vi "pco.camera_Live_ConvertSettings_Example_IMAQ.vi"() -> ()   [LabVIEW 2019]
doc: "A short program to demonstrate the fundamentals of control and image acquision with the pco.camera series. The program records a sequence of images, with \"live\" updating, until the \"StopRecording\" button is pressed. Use ctrl-H for more help on the individual controls and indicators.\n\nCopyright 2004, 2010 The Cooke Corporation."
uses:
  pco.camera/Camera.lvclass
  pco.sdk/TimingControl/TimingControl.lvlib
panel:
  in  "settingsChanged":bool
  in  "Trigger":bool
  in  "LUT File":path
  in  "data_format":T1(ring)=enum."RGBA8"
  out "Image":T2(plugin-control)
  in  "Auto Range":bool
  out "rawImage":u16[][](array[numeric])
  in  "iContrast [%]":i32 min=-100 max=99 step=1
  in  "Gamma":dbl=1.0 min=0.01 max=10.0 step=0.01 format="%.2f"
  in  "whiteBalance":bool
  in  "iScale_max":u16=60000 step=1
  in  "iScale_min":u16=200 step=1
  in  "Image Index":u32 max=9
  out "Recorded Images":u32
  in  "TriggerMode":T3(ring)
  in  "Quit":bool
  out "Error":errorcluster {"code" format="%x"}
  in  "Stop Record":bool
  out "Recording On":bool
  in  "roiY1":u64=2 min=1 max=2160 step=1
  in  "roiX1":u64=2 min=1 max=2560 step=1
  in  "roiY0":u64=1 min=1 max=2159 step=1
  in  "roiX0":u64=1 min=1 max=2559 step=1
  out "Image Height":u64
  out "Image Width":u64
  in  "dwImgCount":u32=10 caption="Required Number of Images" max=2397
  in  "Exposure Time [s]":dbl=0.010000000000000002 min=0.0005 max=2.0 step=0.001
  # "This example demonstrates the image acquisition with one camera in ring buffer mode together with a live display of the latest images during record. After record is stopped, the images can be addressed by index.\nAdditionally the image convert settings can be adjusted at any time\nNote that this example will not be fail save, i.e. doesnt react on errors, just handles them forward to the end\n\nUsage:\nSelect your required image count and the camera setup before you start the program.\nOnce started, the camera class will be initialized and images will be recorded and displayed automatically\nYou can stop the images by pressing stop record.\nAfter stopped, the image at the selected index will be read out\nTo finish the program click on quit application, this will force an exit of the camera class\nYou can change your required ROI after and also during the record."
  # "pco.labview"
  # "Camera Setup"
  # "Recording Control"
  # "Parameters for image readout"
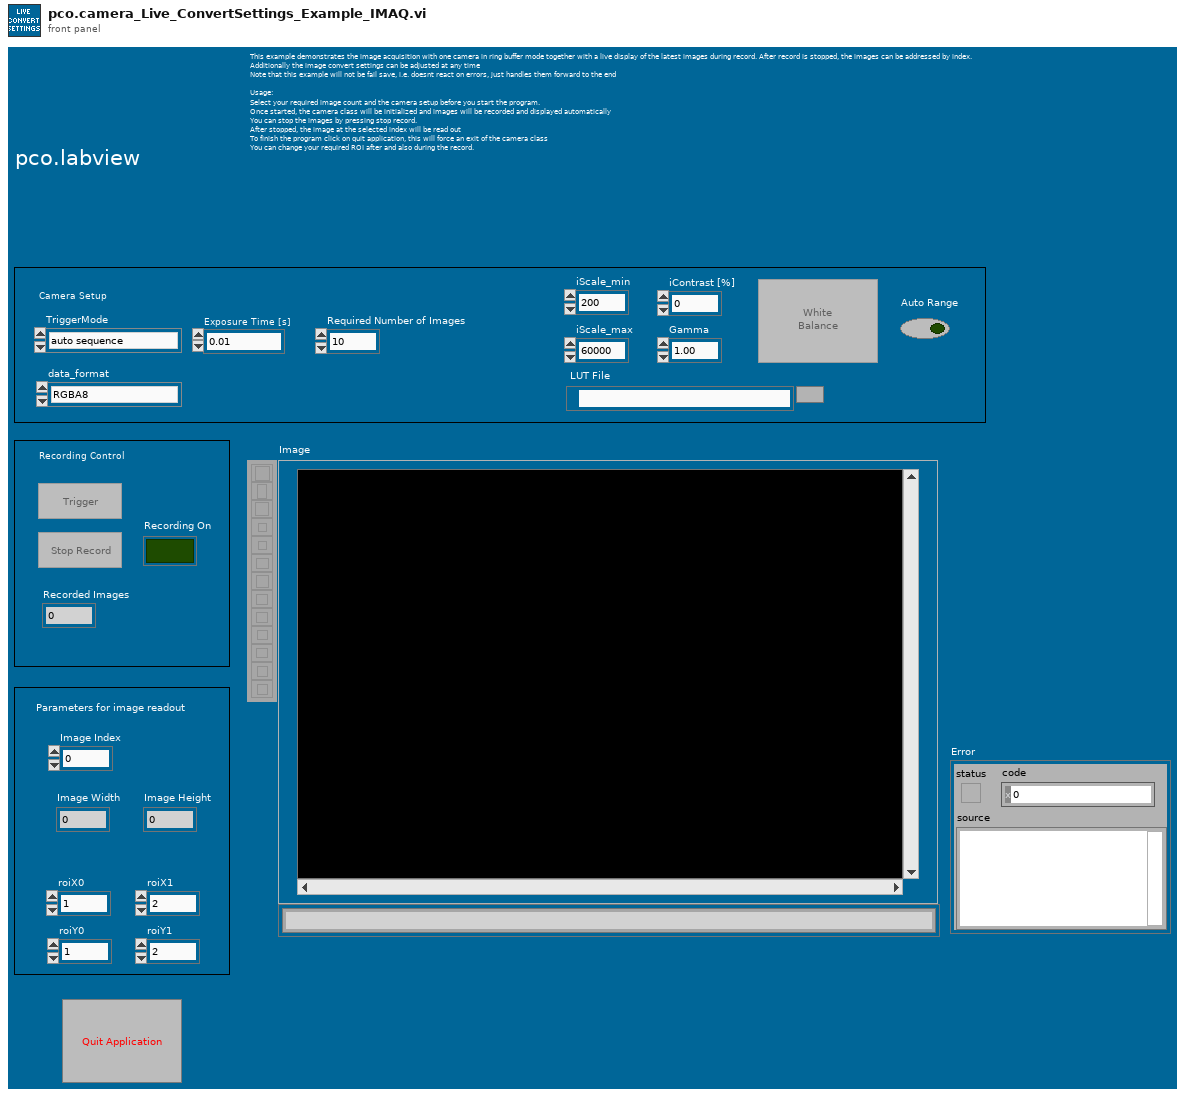
[diagram p1: front panel]
types:
  T1 = enum16{"Undefined", "Mono8", "Mono16", "BGRA8", "RGBA8", "BGRA16", "RGBA16", "CompressedMono8"}
  T2 = typedef "IMAQ Image.ctl" = refnum<image>
  T3 = enum16{"auto sequence", "software trigger", "external exposure start", "external exposure control"}
  T4 = enum16{"sequence", "sequence non blocking", "ring buffer", "fifo", "sequence_dpcore", "sequence_non_blocking_dpcore", "ring_buffer_dpcore", "fifo_dpcore", "tif", "multitif", "pcoraw", "b16", "dicom", "multidicom"}
  T5 = enum8{"Enabled", "Disabled", "Disabled and Grayed Out"}
  T6 = cluster{"serial":u32, "type":u16, "sub_type":u16, "interface_type":u16, "min_exposure_time_s":dbl, "max_exposure_time_s":dbl, "min_exposure_step_s":dbl, "min_delay_time_s":dbl, "max_delay_time_s":dbl, "min_delay_step_s":dbl, "min_width":u64, "min_height":u64, "max_width":u64, "max_height":u64, "roi_step_horz":u64, "roi_step_vert":u64, "roi_symmetric_horz":bool, "roi_symmetric_vert":bool, "has_timestamp_mode":bool, "has_timestamp_mode_ascii_only":bool, "pixelrate_vec":u32[], "has_acquire_mode":bool, "has_ext_acquire_mode":bool, "has_metadata_mode":bool, "has_ram":bool, "binning_horz_vec":u16[], "binning_vert_vec":u16[]}
  T7 = typedef "Image Type" = u32
  T8 = typedef "Camera.lvclass/binning.ctl" = cluster{"vert":u16, "horz":u16}
  T9 = cluster{"exposure_time_s":dbl, "delay_time_s":dbl, "roi":cluster{"x0":u64, "y0":u64, "x1":u64, "y1":u64}, "timestamp_mode":u16, "pixelrate":u32, "trigger_mode":u16, "acquire_mode":u16, "metadata_mode":u16, "noisefilter_mode":u16, "binning":T8}
  T10 = cluster{"sharpen":bool, "adaptive_sharpen":bool, "flip_vertical":bool, "auto_minmax":bool, "min_limit":u16, "max_limit":u16, "gamma":dbl, "contrast":i32, "pco_debayer_algorithm":bool, "color_temperature":i32, "color_saturation":i32, "color_vibrance":i32, "color_tint":i32, "lut_file":path}
  T11 = typedef "Color (U64)" = cluster{"Plane 3 (Blue)":u16, "Plane 2 (Green)":u16, "Plane 1 (Red)":u16, "Plane 4 (alpha)":u16}
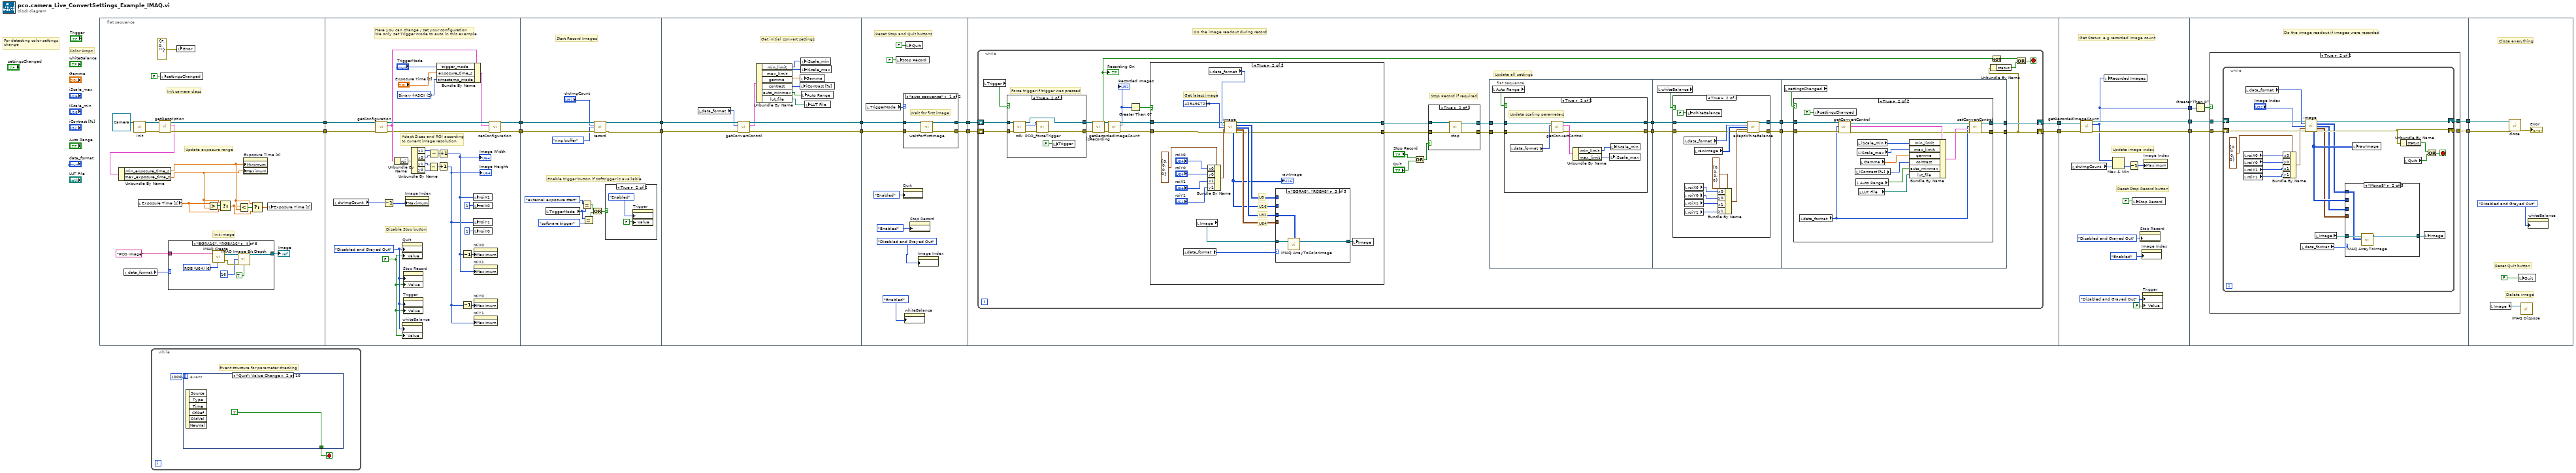
[diagram p0: block diagram]
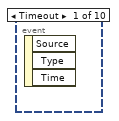
[diagram p2: hidden frame]
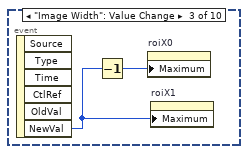
[diagram p3: hidden frame]
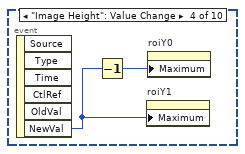
[diagram p4: hidden frame]
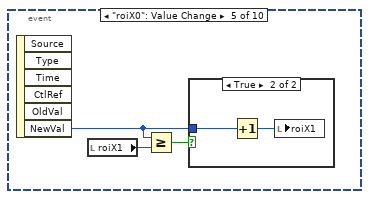
[diagram p5: hidden frame]
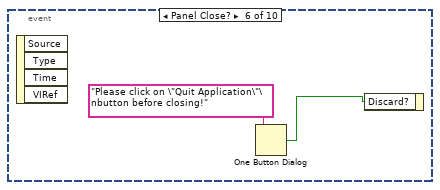
[diagram p7: hidden frame]
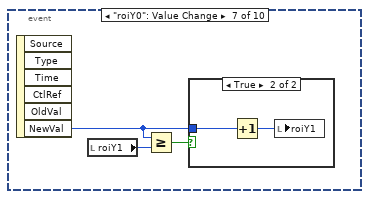
[diagram p8: hidden frame]
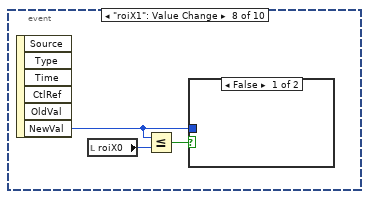
[diagram p10: hidden frame]
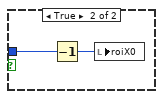
[diagram p11: hidden frame]
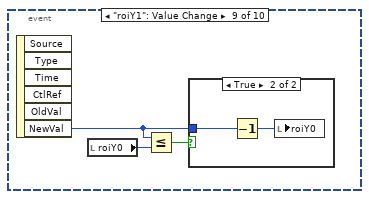
[diagram p12: hidden frame]
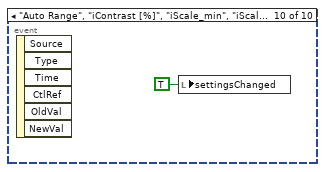
[diagram p14: hidden frame]
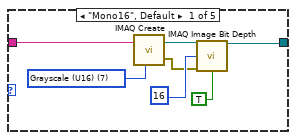
[diagram p15: hidden frame]
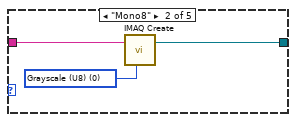
[diagram p16: hidden frame]
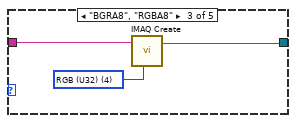
[diagram p17: hidden frame]
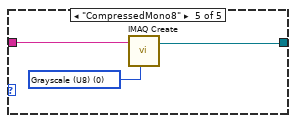
[diagram p18: hidden frame]
diagram:
  # "For detecting color settings\nchange"
  # "Color Props"
  n1 = flat-sequence {
    tunnel: [w24] -> w7
    tunnel: [w23] -> w6
    tunnel: [w63] -> w17
    tunnel: [w67] -> w16
    tunnel: w7 -> [w62]
    tunnel: w6 -> [w61]
    tunnel: w17 -> [w97]
    tunnel: w16 -> [w98]
    tunnel: [w94] -> w11
    tunnel: [w95] -> w8
    tunnel: w11 -> [w111]
    tunnel: [w106] -> w10
    tunnel: [w112] -> w9
    tunnel: w8 -> [w102]
    tunnel: w10 -> [w119]
    tunnel: w9 -> [w120]
    tunnel: [w118] -> w15
    tunnel: [w115] -> w2
    tunnel: w15 -> [w133]
    tunnel: [w132] -> w14
    tunnel: [w131] -> w5
    tunnel: w2 -> [w130]
    tunnel: w14 -> [w280]
    tunnel: [w278] -> w13
    tunnel: w5 -> [w273]
    tunnel: [w272] -> w4
    tunnel: [w271] -> w1
    tunnel: w13 -> [w289]
    tunnel: [w288] -> w12
    tunnel: w4 -> [w287]
    tunnel: [w286] -> w3
    tunnel: w1 -> [w284]
    tunnel: w12 -> [w337]
    tunnel: w3 -> [w334]
    frame #0 {
      # "Init image"
      # "Init camera class"
      # "Update exposure range"
      n2 = local read "data_format"() -> (w19:T1)
      n3 = call-dynamic "init.vi"("Camera in"=refnum<class "Camera.lvclass"> refnum) -> ("Camera out"=w25:refnum<class "Camera.lvclass">, "error out"=w26:errorcluster)  [unwired: 8 in]
      n4 = local read "Exposure Time [s]"() -> (w34:dbl)
      n5 = call-dynamic "getDescription.vi"("error in (no error)"=w26, "Camera in"=w25) -> ("error out"=w23:errorcluster, "description"=w22:T6, "Camera out"=w24:refnum<class "Camera.lvclass">)  [unwired: 7 in]
      n6 = Unbundle By Name(w22) -> ("min_exposure_time_s"=w21:dbl, "max_exposure_time_s"=w20:dbl)
      n7 = local write "settingsChanged"(FALSE ("settingsChanged")) -> ()
      n8 = case shown="\"BGRA16\", \"RGBA16\"" w19 {
        tunnel: "PCO Image" ("Image Name") -> [w41 w45 w47 w54 w57]
        tunnel: [w36 w43 w46 w49 w56] -> w27
        frame "Mono16", Default {
          w42 = T7 7 items=["Grayscale (U8)", "Grayscale (I16)", "Grayscale (SGL)", "Complex (CSG)", "RGB (U32)", "HSL (U32)", "RGB (U64)", "Grayscale (U16)"] ("Image Type")
          n9 = call "IMAQ Create"("Image Name"=w41, "Image Type"=w42) -> ("New Image"=w38:T2, "error out"=w37:errorcluster)  [unwired: 3 in]
          n10 = call "IMAQ Image Bit Depth"("Image"=w38, "Bit Depth (0)"=u32 16, "error in (no error)"=w37, "Get/Set Bit Depth? (Set)"=TRUE) -> ("Image Out"=w36:T2)  [unwired: 9 in, 2 out]
        }
        frame "Mono8" {
          w44 = T7 0 items=["Grayscale (U8)", "Grayscale (I16)", "Grayscale (SGL)", "Complex (CSG)", "RGB (U32)", "HSL (U32)", "RGB (U64)", "Grayscale (U16)"] ("Image Type")
          n11 = call "IMAQ Create"("Image Name"=w45, "Image Type"=w44) -> ("New Image"=w43:T2)  [unwired: 3 in, 1 out]
        }
        frame "BGRA8", "RGBA8" {
          w48 = T7 4 items=["Grayscale (U8)", "Grayscale (I16)", "Grayscale (SGL)", "Complex (CSG)", "RGB (U32)", "HSL (U32)", "RGB (U64)", "Grayscale (U16)"] ("Image Type")
          n12 = call "IMAQ Create"("Image Name"=w47, "Image Type"=w48) -> ("New Image"=w46:T2)  [unwired: 3 in, 1 out]
        }
        frame "BGRA16", "RGBA16" {
          w55 = T7 6 items=["Grayscale (U8)", "Grayscale (I16)", "Grayscale (SGL)", "Complex (CSG)", "RGB (U32)", "HSL (U32)", "RGB (U64)", "Grayscale (U16)"] ("Image Type")
          n13 = call "IMAQ Create"("Image Name"=w54, "Image Type"=w55) -> ("New Image"=w51:T2, "error out"=w50:errorcluster)  [unwired: 3 in]
          n14 = call "IMAQ Image Bit Depth"("Image"=w51, "Bit Depth (0)"=u32 16, "error in (no error)"=w50, "Get/Set Bit Depth? (Set)"=TRUE) -> ("Image Out"=w49:T2)  [unwired: 9 in, 2 out]
        }
        frame "CompressedMono8" {
          w58 = T7 0 items=["Grayscale (U8)", "Grayscale (I16)", "Grayscale (SGL)", "Complex (CSG)", "RGB (U32)", "HSL (U32)", "RGB (U64)", "Grayscale (U16)"] ("Image Type")
          n15 = call "IMAQ Create"("Image Name"=w57, "Image Type"=w58) -> ("New Image"=w56:T2)  [unwired: 3 in, 1 out]
        }
      }
      "Image" <- w27
      n16 = local write "Error"(errorcluster {"status"=FALSE, "code"=0, "source"=""} ("error IO")) -> ()
      n17 = Greater?(x=w34, y=w20) -> (0:w35:bool)
      n18 = Select(t=w20, s=w35, f=w34) -> (s? t:f=w32:dbl)
      n19 = Less?(x=w32, y=w21) -> (x < y?=w33:bool)
      n20 = property on="Exposure Time [s]" class="DigNum (strict)"("Minimum"=w21, "Maximum"=w20) -> ()  [unwired: 2 in, 2 out]
      n21 = Select(t=w21, s=w33, f=w32) -> (s? t:f=w31:dbl)
      n22 = local write "Exposure Time [s]"(w31) -> ()
    }
    frame #1 {
      w73 = u16 2 items=["OFF", "Binary", "Binary+ASCII", "ASCII"] ("wTimeStampMode")
      w59 = FALSE ("Stop")
      w60 = T5."Disabled and Grayed Out" ("Disabled")
      # "Disable Stop button"
      # "Adapt Sizes and ROI according\nto current image resolution"
      # "Here you can change / set your configuration\nWe only set Trigger mode to auto in this example"
      n23 = local read "dwImgCount"() -> (w74:u32)
      n24 = call-dynamic "getConfiguration.vi"("error in (no error)"=w61, "Camera in"=w62) -> ("error out"=w68:errorcluster, "configuration"=w79:T9, "Camera out"=w70:refnum<class "Camera.lvclass">)  [unwired: 7 in]
      n25 = Decrement(x=w74) -> (x-1=w64:u32)
      n26 = Unbundle By Name(w79) -> ("roi"=w80:cluster{"x0":u64, "y0":u64, "x1":u64, "y1":u64})
      n27 = property on="Quit" class="Bool (strict)"("DisabledEnum"=w60, "Value"=w59) -> ()  [unwired: 2 in, 2 out]
      n28 = property on="whiteBalance" class="Bool (strict)"("DisabledEnum"=w60, "Value"=w59) -> ()  [unwired: 2 in, 2 out]
      n29 = property on="Stop Record" class="Bool (strict)"("DisabledEnum"=w60, "Value"=w59) -> ()  [unwired: 2 in, 2 out]
      n30 = property on="Trigger" class="Bool (strict)"("DisabledEnum"=w60, "Value"=w59) -> ()  [unwired: 2 in, 2 out]
      n31 = property on="Image Index" class="DigNum (strict)"("Maximum"=w64) -> ()  [unwired: 2 in, 2 out]
      n32 = Unbundle By Name(w80) -> ("x1"=w82:u64, "x0"=w81:u64, "y1"=w84:u64, "y0"=w83:u64)
      n33 = Subtract(x=w84, y=w83) -> (x-y=w86:u64)
      n34 = Subtract(x=w82, y=w81) -> (x-y=w85:u64)
      n35 = Bundle By Name(cluster=w79, "trigger_mode"="TriggerMode", "exposure_time_s"="Exposure Time [s]", "timestamp_mode"=w73) -> (w69:T9)
      n36 = Increment(x=w86) -> (x+1=w65:u64)
      "Image Height" <- w65
      n37 = Increment(x=w85) -> (x+1=w66:u64)
      "Image Width" <- w66
      n38 = Decrement(x=w66) -> (x-1=w77:u64)
      n39 = Decrement(x=w65) -> (x-1=w78:u64)
      n40 = local write "roiX1"(w66) -> ()
      n41 = local write "roiX0"(u64 1 ("roiY0")) -> ()
      n42 = local write "roiY1"(w65) -> ()
      n43 = local write "roiY0"(u64 1 ("roiY0")) -> ()
      n44 = property on="roiX0" class="DigNum (strict)"("Maximum"=w77) -> ()  [unwired: 2 in, 2 out]
      n45 = property on="roiX1" class="DigNum (strict)"("Maximum"=w66) -> ()  [unwired: 2 in, 2 out]
      n46 = property on="roiY0" class="DigNum (strict)"("Maximum"=w78) -> ()  [unwired: 2 in, 2 out]
      n47 = property on="roiY1" class="DigNum (strict)"("Maximum"=w65) -> ()  [unwired: 2 in, 2 out]
      n48 = call-dynamic "setConfiguration.vi"("error in (no error)"=w68, "configuration"=w69, "Camera in"=w70) -> ("error out"=w67:errorcluster, "Camera out"=w63:refnum<class "Camera.lvclass">)  [unwired: 7 in]
    }
    frame #2 {
      # "Enable trigger button if softtrigger is available"
      # "Start Record Images"
      n49 = local read "TriggerMode"() -> (w92:T3)
      n50 = Equal?(x=T3."external exposure start" ("TriggerMode"), y=w92) -> (x = y?=w89:bool)
      n51 = Equal?(x=w92, y=T3."software trigger" ("TriggerMode")) -> (x = y?=w88:bool)
      n52 = Or(x=w89, y=w88) -> (x .or. y?=w90:bool)
      n53 = call-dynamic "record.vi"("Camera in"=w97, "num_images"="dwImgCount", "record_mode"=T4."ring buffer", "error in (no error)"=w98) -> ("Camera out"=w95:refnum<class "Camera.lvclass">, "error out"=w94:errorcluster)  [unwired: 10 in]
      n54 = case shown="True" w90 {
        frame False {
        }
        frame True {
          n55 = property on="Trigger" class="Bool (strict)"("DisabledEnum"=T5."Enabled" ("Disabled"), "Value"=FALSE ("Trigger")) -> ()  [unwired: 2 in, 2 out]
        }
      }
    }
    frame #3 {
      # "Get initial convert settings"
      n56 = local read "data_format"() -> (w101:T1)
      n57 = call-dynamic "getConvertControl.vi"("error in (no error)"=w111, "data_format"=w101, "Camera in"=w102) -> ("error out"=w106:errorcluster, "convert_control"=w110:T10, "Camera out"=w112:refnum<class "Camera.lvclass">)  [unwired: 6 in]
      n58 = Unbundle By Name(w110) -> ("min_limit"=w108:u16, "max_limit"=w107:u16, "gamma"=w109:dbl, "contrast"=w105:i32, "auto_minmax"=w104:bool, "lut_file"=w103:path)
      n59 = local write "iContrast [%]"(w105) -> ()
      n60 = local write "Gamma"(w109) -> ()
      n61 = local write "iScale_min"(w108) -> ()
      n62 = local write "iScale_max"(w107) -> ()
      n63 = local write "Auto Range"(w104) -> ()
      n64 = local write "LUT File"(w103) -> ()
    }
    frame #4 {
      # "Reset Stop and Quit buttons"
      n65 = local read "TriggerMode"() -> (w113:T3)
      n66 = local write "Stop Record"(FALSE ("Stop Record")) -> ()
      n67 = case shown="\"auto sequence\"" w113 {
        tunnel: w120 -> [w127 w129]
        tunnel: w119 -> [w126 w128]
        tunnel: [w125 w128] -> w118
        tunnel: [w124 w129] -> w115
        frame "auto sequence" {
          # "Wait for first image"
          n68 = call-dynamic "waitForFirstImage.vi"("error in (no error)"=w126, "Camera in"=w127) -> ("error out"=w125:errorcluster, "Camera out"=w124:refnum<class "Camera.lvclass">)  [unwired: 8 in]
        }
        frame Default {
          # "Don't wait \nif we trigger"
        }
      }
      n69 = property on="Quit" class="Bool (strict)"("DisabledEnum"=T5."Enabled" ("Disabled")) -> ()  [unwired: 2 in, 2 out]
      n70 = property on="whiteBalance" class="Bool (strict)"("DisabledEnum"=T5."Enabled" ("Disabled")) -> ()  [unwired: 2 in, 2 out]
      n71 = local write "Quit"(FALSE ("Stop")) -> ()
      n72 = property on="Stop Record" class="Bool (strict)"("DisabledEnum"=T5."Enabled" ("Disabled")) -> ()  [unwired: 2 in, 2 out]
      n73 = property on="Image Index" class="DigNum (strict)"("DisabledEnum"=T5."Disabled and Grayed Out" ("Disabled")) -> ()  [unwired: 2 in, 2 out]
    }
    frame #5 {
      # "Do the image readout during record"
      n74 = while {
        shift-right: [w143] -> w132
        shift-left: w133 -> [w146]
        shift-right: [w149] -> w131
        shift-left: w130 -> [w147]
        stop <- w161 stop-if-true
        # "Stop Record if required"
        # "Force trigger if trigger was pressed"
        # "Update all settings"
        n75 = local read "Trigger"() -> (w148:bool)
        n76 = case shown="True" w148 {
          tunnel: w147 -> [w205 w210]
          tunnel: w146 -> [w204 w209]
          tunnel: [w205 w208] -> w145
          tunnel: [w204 w207] -> w144
          frame False {
          }
          frame True {
            n77 = call-dynamic "sdk.vi"("Camera in"=w210, "error in (no error)"=w209) -> ("Camera out"=w208:refnum<class "Camera.lvclass">, "sdk"=w211:u64, "error out"=w212:errorcluster)  [unwired: 11 in]
            n78 = call "PCO_ForceTrigger.vi"("error in (no error)"=w212, "ph"=w211) -> ("error out"=w207:errorcluster)  [unwired: 6 in, 3 out]
            n79 = local write "Trigger"(FALSE ("Trigger")) -> ()
          }
        }
        n80 = call-dynamic "isRecording.vi"("Camera in"=w145, "error in (no error)"=w144) -> ("Camera out"=w157:refnum<class "Camera.lvclass">, "recording"=w159:bool, "error out"=w156:errorcluster)  [unwired: 11 in]
        "Recording On" <- w159
        n81 = call-dynamic "getRecordedImageCount.vi"("Camera in"=w157, "error in (no error)"=w156) -> ("Camera out"=w154:refnum<class "Camera.lvclass">, "recorded_image_count"=w142:u32, "error out"=w155:errorcluster)  [unwired: 11 in]
        "Recorded Images" <- w142
        n82 = Greater Than 0?(x=w142) -> (x > 0?=w141:bool)
        n83 = case shown="True" w141 {
          tunnel: w155 -> [w168 w181]
          tunnel: w154 -> [w169 w172]
          tunnel: [w168 w170] -> w137
          tunnel: [w169 w171] -> w136
          frame False {
          }
          frame True {
            # "U64"
            # "U32"
            # "U8"
            # "U16"
            # "Get latest image"
            n84 = local read "data_format"() -> (w173:T1)
            n85 = local read "Image"() -> (w178:T2)
            n86 = Bundle By Name(cluster=cluster{"x0":u64, "y0":u64, "x1":u64, "y1":u64} {"x0"=0, "y0"=0, "x1"=0, "y1"=0} ("roi"), "x0"="roiX0", "y0"="roiY0", "x1"="roiX1", "y1"="roiY1") -> (w184:cluster{"x0":u64, "y0":u64, "x1":u64, "y1":u64})
            n87 = local read "data_format"() -> (w180:T1)
            n88 = call-dynamic "image.vi"("Camera in"=w172, "data_format"=w180, "image_index"=u32 4294967295 ("dwImgIdx"), "roi"=w184, "error in (no error)"=w181) -> ("Camera out"=w171:refnum<class "Camera.lvclass">, "image (U8)"=w175:u8[][], "image (U32)"=w176:u32[][], "image (U64)"=w177:T11[][], "raw_image (U16)"=w174:u16[][], "error out"=w170:errorcluster)  [unwired: 3 in, 2 out]
            "rawImage" <- w174
            n89 = case shown="\"BGRA8\", \"RGBA8\"" w173 {
              tunnel: w178 -> [w191 w194 w197 w200 w203]
              tunnel: [w189 w192 w196 w198 w202] -> w179
              tunnel: w177 -> [_ _ _ w199 _]
              tunnel: w176 -> [_ _ w195 _ _]
              tunnel: w175 -> [_ w193 _ _ w201]
              tunnel: w174 -> [w190 _ _ _ _]
              frame "Mono16", Default {
                n90 = call "IMAQ ArrayToImage"("Image Pixels (U16)"=w190, "Image"=w191) -> ("Image Out"=w189:T2)  [unwired: 8 in, 1 out]
              }
              frame "Mono8" {
                n91 = call "IMAQ ArrayToImage"("Image Pixels (U8)"=w193, "Image"=w194) -> ("Image Out"=w192:T2)  [unwired: 8 in, 1 out]
              }
              frame "BGRA8", "RGBA8" {
                n92 = call "IMAQ ArrayToColorImage"("Image Pixels (U32)"=w195, "Image"=w197) -> ("Image Out"=w196:T2)  [unwired: 3 in, 1 out]
              }
              frame "BGRA16", "RGBA16" {
                n93 = call "IMAQ ArrayToColorImage"("Image"=w200, "Image Pixels (U64)"=w199) -> ("Image Out"=w198:T2)  [unwired: 3 in, 1 out]
              }
              frame "CompressedMono8" {
                n94 = call "IMAQ ArrayToImage"("Image Pixels (U8)"=w201, "Image"=w203) -> ("Image Out"=w202:T2)  [unwired: 8 in, 1 out]
              }
            }
            n95 = local write "Image"(w179) -> ()
          }
        }
        n96 = Or(x="Stop Record", y="Quit") -> (x .or. y?=w140:bool)
        n97 = case shown="True" w140 {
          tunnel: w137 -> [w163 w164]
          tunnel: [w162 w166] -> w135
          tunnel: [w163 w167] -> w134
          tunnel: w136 -> [w162 w165]
          frame False {
          }
          frame True {
            n98 = call-dynamic "stop.vi"("error in (no error)"=w164, "Camera in"=w165) -> ("error out"=w167:errorcluster, "Camera out"=w166:refnum<class "Camera.lvclass">)  [unwired: 8 in]
          }
        }
        n99 = flat-sequence {
          tunnel: w134 -> [w215]
          tunnel: w135 -> [w216]
          tunnel: [w214] -> w153
          tunnel: [w213] -> w152
          tunnel: w153 -> [w231]
          tunnel: w152 -> [w230]
          tunnel: [w229] -> w151
          tunnel: [w228] -> w150
          tunnel: w151 -> [w250]
          tunnel: w150 -> [w251]
          tunnel: [w249] -> w143
          tunnel: [w248] -> w149
          frame #0 {
            n100 = local read "Auto Range"() -> (w217:bool)
            n101 = case shown="True" w217 {
              tunnel: w216 -> [w219 w223]
              tunnel: w215 -> [w218 w222]
              tunnel: [w218 w221] -> w214
              tunnel: [w219 w220] -> w213
              frame False {
              }
              frame True {
                # "Update scaling parameters"
                n102 = local read "data_format"() -> (w227:T1)
                n103 = call-dynamic "getConvertControl.vi"("error in (no error)"=w222, "data_format"=w227, "Camera in"=w223) -> ("error out"=w221:errorcluster, "convert_control"=w224:T10, "Camera out"=w220:refnum<class "Camera.lvclass">)  [unwired: 6 in]
                n104 = Unbundle By Name(w224) -> ("min_limit"=w225:u16, "max_limit"=w226:u16)
                n105 = local write "iScale_max"(w226) -> ()
                n106 = local write "iScale_min"(w225) -> ()
              }
            }
          }
          frame #1 {
            n107 = local read "whiteBalance"() -> (w232:bool)
            n108 = case shown="True" w232 {
              tunnel: w231 -> [w233 w239]
              tunnel: w230 -> [w234 w238]
              tunnel: [w233 w237] -> w229
              tunnel: [w234 w236] -> w228
              frame False {
              }
              frame True {
                n109 = local read "data_format"() -> (w246:T1)
                n110 = local read "roiX0"() -> (w244:u64)
                n111 = local read "roiY0"() -> (w243:u64)
                n112 = local read "roiX1"() -> (w242:u64)
                n113 = local read "roiY1"() -> (w235:u64)
                n114 = local write "whiteBalance"(FALSE ("whiteBalance")) -> ()
                n115 = local read "rawImage"() -> (w245:u16[][])
                n116 = Bundle By Name(cluster=cluster{"x0":u64, "y0":u64, "x1":u64, "y1":u64} {"x0"=0, "y0"=0, "x1"=0, "y1"=0} ("roi"), "x0"=w244, "y0"=w243, "x1"=w242, "y1"=w235) -> (w241:cluster{"x0":u64, "y0":u64, "x1":u64, "y1":u64})
                n117 = call-dynamic "adaptWhiteBalance.vi"("Camera in"=w238, "data_format"=w246, "raw_image (U16)"=w245, "roi"=w241, "error in (no error)"=w239) -> ("Camera out"=w236:refnum<class "Camera.lvclass">, "error out"=w237:errorcluster)  [unwired: 9 in]
              }
            }
          }
          frame #2 {
            n118 = local read "settingsChanged"() -> (w252:bool)
            n119 = case shown="True" w252 {
              tunnel: w251 -> [w254 w260]
              tunnel: w250 -> [w253 w259]
              tunnel: [w253 w256] -> w249
              tunnel: [w254 w255] -> w248
              frame False {
              }
              frame True {
                n120 = local read "data_format"() -> (w258:T1)
                n121 = local write "settingsChanged"(FALSE ("whiteBalance")) -> ()
                n122 = call-dynamic "getConvertControl.vi"("error in (no error)"=w259, "data_format"=w258, "Camera in"=w260) -> ("error out"=w262:errorcluster, "convert_control"=w269:T10, "Camera out"=w263:refnum<class "Camera.lvclass">)  [unwired: 6 in]
                n123 = local read "iContrast [%]"() -> (w265:i32)
                n124 = local read "Auto Range"() -> (w264:bool)
                n125 = local read "iScale_max"() -> (w267:u16)
                n126 = local read "iScale_min"() -> (w268:u16)
                n127 = local read "LUT File"() -> (w257:path)
                n128 = local read "Gamma"() -> (w266:dbl)
                n129 = Bundle By Name(cluster=w269, "min_limit"=w268, "max_limit"=w267, "gamma"=w266, "contrast"=w265, "auto_minmax"=w264, "lut_file"=w257) -> (w261:T10)
                n130 = call-dynamic "setConvertControl.vi"("error in (no error)"=w262, "convert_control"=w261, "data_format"=w258, "Camera in"=w263) -> ("error out"=w256:errorcluster, "Camera out"=w255:refnum<class "Camera.lvclass">)  [unwired: 6 in]
              }
            }
          }
        }
        n131 = Unbundle By Name(w143) -> ("status"=w160:bool)
        n132 = Not(x=w159) -> (.not. x?=w158:bool)
        n133 = Or(x=w158, y=w160) -> (x .or. y?=w161:bool)
      }
    }
    frame #6 {
      # "Update image index"
      # "Reset Stop Record button"
      # "Get Status, e.g recorded image count"
      n134 = local read "dwImgCount"() -> (w279:u32)
      n135 = call-dynamic "getRecordedImageCount.vi"("Camera in"=w273, "error in (no error)"=w280) -> ("Camera out"=w272:refnum<class "Camera.lvclass">, "recorded_image_count"=w271:u32, "error out"=w278:errorcluster)  [unwired: 11 in]
      n136 = local write "Recorded Images"(w271) -> ()
      n137 = Max & Min(x=w271, y=w279) -> (min(x,y)=w281:u32)  [unwired: 1 out]
      n138 = Decrement(x=w281) -> (x-1=w276:u32)
      n139 = local write "Stop Record"(FALSE ("Stop Record")) -> ()
      n140 = property on="Stop Record" class="Bool (strict)"("DisabledEnum"=T5."Disabled and Grayed Out" ("Disabled")) -> ()  [unwired: 2 in, 2 out]
      n141 = property on="Image Index" class="DigNum (strict)"("DisabledEnum"=T5."Enabled" ("Disabled")) -> ()  [unwired: 2 in, 2 out]
      n142 = property on="Trigger" class="Bool (strict)"("DisabledEnum"=T5."Disabled and Grayed Out" ("Disabled"), "Value"=FALSE ("Trigger")) -> ()  [unwired: 2 in, 2 out]
      n143 = property on="Image Index" class="DigNum (strict)"("Maximum"=w276) -> ()  [unwired: 2 in, 2 out]
    }
    frame #7 {
      # "Do the image readout if images were recorded"
      n144 = Greater Than 0?(x=w284) -> (x > 0?=w285:bool)
      n145 = case shown="True" w285 {
        tunnel: w289 -> [w290 w295]
        tunnel: [w290 w294] -> w288
        tunnel: w287 -> [w291 w293]
        tunnel: [w291 w292] -> w286
        frame False {
        }
        frame True {
          n146 = while {
            shift-right: [w309] -> w294
            shift-left: w295 -> [w317]
            shift-right: [w296] -> w292
            shift-left: w293 -> [w297]
            stop <- w311 stop-if-true
            n147 = local read "roiX0"() -> (w307:u64)
            n148 = local read "roiY0"() -> (w308:u64)
            n149 = local read "roiX1"() -> (w315:u64)
            n150 = local read "roiY1"() -> (w314:u64)
            n151 = local read "data_format"() -> (w305:T1)
            n152 = Bundle By Name(cluster=cluster{"x0":u64, "y0":u64, "x1":u64, "y1":u64} {"x0"=0, "y0"=0, "x1"=0, "y1"=0} ("roi"), "x0"=w307, "y0"=w308, "x1"=w315, "y1"=w314) -> (w316:cluster{"x0":u64, "y0":u64, "x1":u64, "y1":u64})
            n153 = local read "data_format"() -> (w298:T1)
            n154 = call-dynamic "image.vi"("Camera in"=w297, "data_format"=w305, "image_index"="Image Index", "roi"=w316, "error in (no error)"=w317) -> ("Camera out"=w296:refnum<class "Camera.lvclass">, "image (U8)"=w301:u8[][], "image (U32)"=w300:u32[][], "image (U64)"=w299:T11[][], "raw_image (U16)"=w302:u16[][], "error out"=w309:errorcluster)  [unwired: 3 in, 2 out]
            n155 = local read "Image"() -> (w303:T2)
            n156 = case shown="\"Mono8\"" w298 {
              tunnel: w303 -> [w320 w323 w326 w329 w332]
              tunnel: [w318 w321 w325 w327 w331] -> w304
              tunnel: w299 -> [_ _ _ w328 _]
              tunnel: w300 -> [_ _ w324 _ _]
              tunnel: w301 -> [_ w322 _ _ w330]
              tunnel: w302 -> [w319 _ _ _ _]
              frame "Mono16", Default {
                n157 = call "IMAQ ArrayToImage"("Image Pixels (U16)"=w319, "Image"=w320) -> ("Image Out"=w318:T2)  [unwired: 8 in, 1 out]
              }
              frame "Mono8" {
                n158 = call "IMAQ ArrayToImage"("Image Pixels (U8)"=w322, "Image"=w323) -> ("Image Out"=w321:T2)  [unwired: 8 in, 1 out]
              }
              frame "BGRA8", "RGBA8" {
                n159 = call "IMAQ ArrayToColorImage"("Image Pixels (U32)"=w324, "Image"=w326) -> ("Image Out"=w325:T2)  [unwired: 3 in, 1 out]
              }
              frame "BGRA16", "RGBA16" {
                n160 = call "IMAQ ArrayToColorImage"("Image"=w329, "Image Pixels (U64)"=w328) -> ("Image Out"=w327:T2)  [unwired: 3 in, 1 out]
              }
              frame "CompressedMono8" {
                n161 = call "IMAQ ArrayToImage"("Image Pixels (U8)"=w330, "Image"=w332) -> ("Image Out"=w331:T2)  [unwired: 8 in, 1 out]
              }
            }
            n162 = local write "rawImage"(w302) -> ()
            n163 = Unbundle By Name(w309) -> ("status"=w312:bool)
            n164 = local read "Quit"() -> (w313:bool)
            n165 = local write "Image"(w304) -> ()
            n166 = Or(x=w312, y=w313) -> (x .or. y?=w311:bool)
          }
        }
      }
    }
    frame #8 {
      # "Delete image"
      # "Close everything"
      # "Reset Quit button"
      n167 = local read "Image"() -> (w333:T2)
      n168 = call-dynamic "close.vi"("error in (no error)"=w337, "Camera in"=w334) -> ("error out"=→"Error":errorcluster)  [unwired: 9 in]
      n169 = local write "Quit"(FALSE ("Stop Record")) -> ()
      n170 = call "IMAQ Dispose"("Image"=w333) -> ()  [unwired: 5 in, 1 out]
      n171 = property on="whiteBalance" class="Bool (strict)"("DisabledEnum"=T5."Disabled and Grayed Out" ("Disabled")) -> ()  [unwired: 2 in, 2 out]
    }
  }
  n172 = while {
    stop <- w339 stop-if-true
    # "Event structure for parameter checking"
    n173 = event shown="[1] \"Quit\": Value Change" {
      selector: _ -> [_ _ _ _ _ _ _ _ _ _]
      dyn-events: _ -> [_ _ _ _ _ _ _ _ _ _]
      timeout: 1000 -> [_ _ _ _ _ _ _ _ _ _]
      tunnel: [_ TRUE _ _ _ _ _ _ _ _] -> w339
      event Timeout {
        n174 = event-data() -> ()  [unwired: 1 in, 3 out]
      }
      event "Quit": Value Change {
        n175 = event-data() -> ()  [unwired: 1 in, 6 out]
      }
      event "Image Width": Value Change {
        n176 = event-data() -> ("NewVal"=w342:u64)  [unwired: 1 in, 5 out]
        n177 = Decrement(x=w342) -> (x-1=w343:u64)
        n178 = property on="roiX0" class="DigNum (strict)"("Maximum"=w343) -> ()  [unwired: 2 in, 2 out]
        n179 = property on="roiX1" class="DigNum (strict)"("Maximum"=w342) -> ()  [unwired: 2 in, 2 out]
      }
      event "Image Height": Value Change {
        n180 = event-data() -> ("NewVal"=w344:u64)  [unwired: 1 in, 5 out]
        n181 = Decrement(x=w344) -> (x-1=w345:u64)
        n182 = property on="roiY1" class="DigNum (strict)"("Maximum"=w344) -> ()  [unwired: 2 in, 2 out]
        n183 = property on="roiY0" class="DigNum (strict)"("Maximum"=w345) -> ()  [unwired: 2 in, 2 out]
      }
      event "roiX0": Value Change {
        n184 = event-data() -> ("NewVal"=w346:u64)  [unwired: 1 in, 5 out]
        n185 = local read "roiX1"() -> (w348:u64)
        n186 = Greater Or Equal?(x=w346, y=w348) -> (x >= y?=w347:bool)
        n187 = case shown="True" w347 {
          tunnel: w346 -> [_ w350]
          frame False {
          }
          frame True {
            n188 = Increment(x=w350) -> (x+1=w349:u64)
            n189 = local write "roiX1"(w349) -> ()
          }
        }
      }
      event Panel Close? {
        n190 = event-data() -> ()  [unwired: 1 in, 4 out]
        n191 = One Button Dialog(message="Please click on \"Quit Application\"\nbutton before closing!") -> (true=w351:bool)  [unwired: 1 in]
        n192 = event-data("Discard?"=w351) -> ()  [unwired: 1 in, 1 out]
      }
      event "roiY0": Value Change {
        n193 = event-data() -> ("NewVal"=w353:u64)  [unwired: 1 in, 5 out]
        n194 = local read "roiY1"() -> (w355:u64)
        n195 = Greater Or Equal?(x=w353, y=w355) -> (x >= y?=w354:bool)
        n196 = case shown="True" w354 {
          tunnel: w353 -> [_ w357]
          frame False {
          }
          frame True {
            n197 = Increment(x=w357) -> (x+1=w356:u64)
            n198 = local write "roiY1"(w356) -> ()
          }
        }
      }
      event "roiX1": Value Change {
        n199 = event-data() -> ("NewVal"=w358:u64)  [unwired: 1 in, 5 out]
        n200 = local read "roiX0"() -> (w360:u64)
        n201 = Less Or Equal?(x=w358, y=w360) -> (x <= y?=w359:bool)
        n202 = case shown="False" w359 {
          tunnel: w358 -> [_ w362]
          frame False {
          }
          frame True {
            n203 = Decrement(x=w362) -> (x-1=w361:u64)
            n204 = local write "roiX0"(w361) -> ()
          }
        }
      }
      event "roiY1": Value Change {
        n205 = event-data() -> ("NewVal"=w363:u64)  [unwired: 1 in, 5 out]
        n206 = local read "roiY0"() -> (w365:u64)
        n207 = Less Or Equal?(x=w363, y=w365) -> (x <= y?=w364:bool)
        n208 = case shown="True" w364 {
          tunnel: w363 -> [_ w367]
          frame False {
          }
          frame True {
            n209 = Decrement(x=w367) -> (x-1=w366:u64)
            n210 = local write "roiY0"(w366) -> ()
          }
        }
      }
      event "Auto Range", "iContrast [%]", "iScale_min", "iScale_max", "Gamma", "LUT File": Value Change {
        n211 = event-data() -> ()  [unwired: 1 in, 6 out]
        n212 = local write "settingsChanged"(TRUE ("settingsChanged")) -> ()
      }
    }
  }
